vi "Move Absolute Motor.vi"(6 "Position (0 units)":dbl min=-2000000000.0 max=2000000000.0 format="%.6f", 7 "timeout":dbl format="%#_13g", 8 "error in (no error)":errorcluster, 9 "Axis (1)":i32=1 min=1 max=3, 10 "VISA resource name":refnum<visa-resource-name>, 11 "ESP301 in":refnum<class "ESP301.lvclass">) -> (0 "error out":errorcluster, 2 "VISA resource name out":refnum<visa-resource-name>, 3 "ESP301 out":refnum<class "ESP301.lvclass">)   [LabVIEW 2020, in "ESP301.lvclass"]
uses:
  ESP301.lvclass
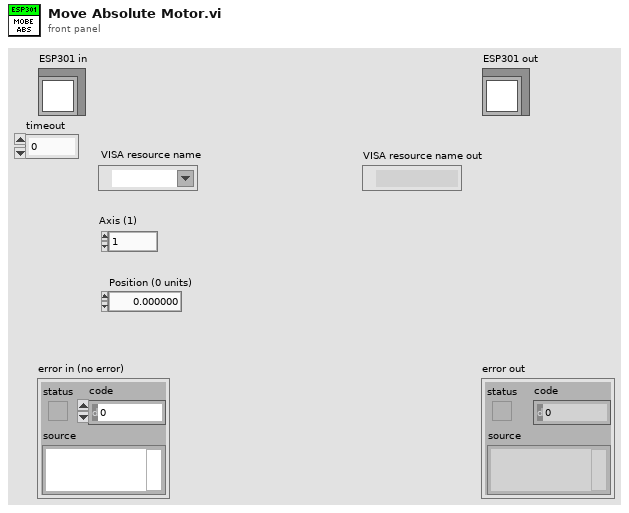
[diagram p1: front panel]
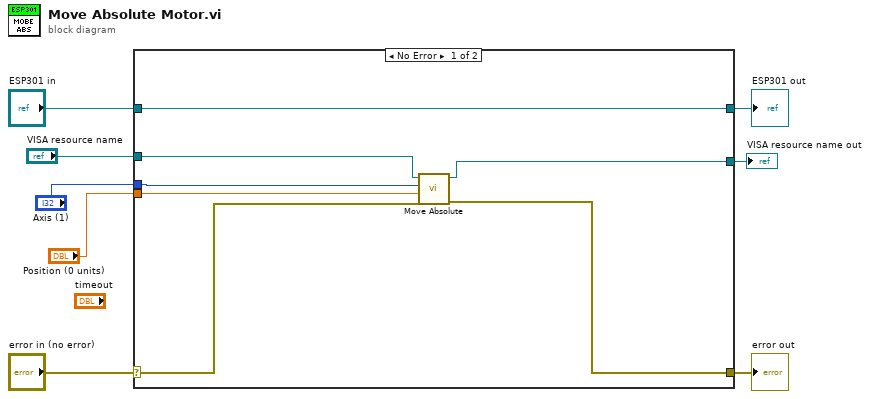
[diagram p0: block diagram]
diagram:
  n1 = case shown="No Error" "error in (no error)" {
    selector: "error in (no error)" -> [w12 w18]
    tunnel: [w11 w18] -> w7
    tunnel: [w15 w17] -> w5
    tunnel: "ESP301 in" -> [w15 w17]
    tunnel: "VISA resource name" -> [w14 w16]
    tunnel: [w13 w16] -> w3
    tunnel: "Position (0 units)" -> [w10 _]
    tunnel: "Axis (1)" -> [w9 _]
    frame No Error {
      n2 = call "Move Absolute.vi"("error in (no error)"=w12, "Position (0 units)"=w10, "Axis (1)"=w9, "VISA resource name"=w14) -> ("error out"=w11:errorcluster, "VISA resource name out"=w13:refnum<visa-resource-name>)  [unwired: 2 in]
    }
    frame Error {
    }
  }
  "error out" <- w7
  "ESP301 out" <- w5
  "VISA resource name out" <- w3
